vi "Initialize.vi"(8 "error in (no error)":errorcluster, 11 "GRMActor in":refnum<class "FlatFieldUI.lvclass">) -> (0 "error out":errorcluster, 3 "GRMActor out":refnum<class "FlatFieldUI.lvclass">)   [LabVIEW 2020, in "FlatField.lvlib" / "FlatFieldUI.lvlib" / "FlatFieldUI.lvclass"]
uses:
  FlatFieldUI.lvclass
  FlatField/FlatField/FlatField Status.ctl
  Displayer/Displayer/FlatField Method.ctl
  FlatFieldUI.lvclass/FlatFieldUI.ctl
  Hardware Abstraction Layer/Component/GenericActor/GenericActor/GenericController.lvclass
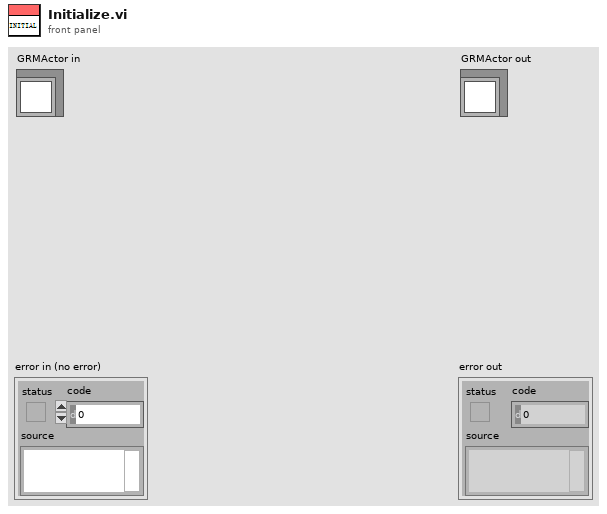
[diagram p1: front panel]
types:
  T1 = typedef "FlatField.lvlib/FlatFieldUI.lvlib/FlatFieldUI.lvclass/FlatField Method.ctl" = i32
  T2 = typedef "Image Type" = u32
  T3 = typedef "FlatField.lvlib/FlatFieldUI.lvlib/FlatFieldUI.lvclass/FlatField Status.ctl" = i32
  T4 = typedef "IMAQ Image.ctl" = refnum<image>
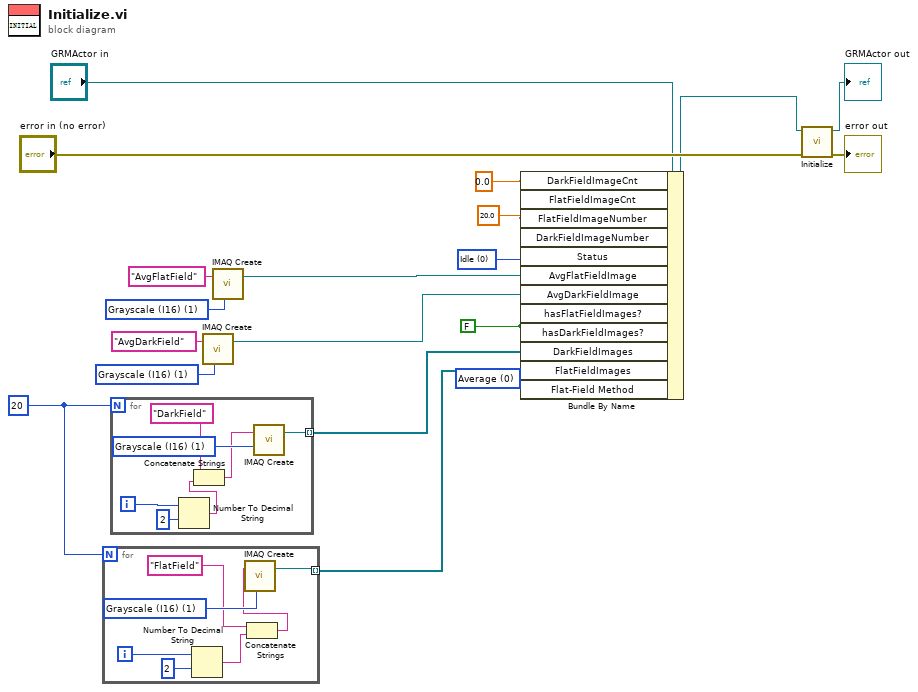
[diagram p0: block diagram]
diagram:
  w3 = T1 0 items=["Average", "Median"] ("Flat-Field Method")
  w6 = 20
  w7 = FALSE ("hasFlatFieldImages?")
  w10 = T2 1 items=["Grayscale (U8)", "Grayscale (I16)", "Grayscale (SGL)", "Complex (CSG)", "RGB (U32)", "HSL (U32)", "RGB (U64)", "Grayscale (U16)"] ("Image Type")
  w11 = T2 1 items=["Grayscale (U8)", "Grayscale (I16)", "Grayscale (SGL)", "Complex (CSG)", "RGB (U32)", "HSL (U32)", "RGB (U64)", "Grayscale (U16)"] ("Image Type")
  w14 = 0.0 ("DarkFieldImageCnt")
  w15 = 20.0 ("FieldFieldImageNumber")
  w16 = T3 0 items=["Idle", "Taking DarkField Images", "Taking FlatField Image", "Doing FlatField", ""] ("Flat-Field Status")
  n1 = for {
    N: w6 -> [_]
    tunnel: [w20] -> w4 mode=indexing
    i -> [w25]
    w26 = T2 1 items=["Grayscale (U8)", "Grayscale (I16)", "Grayscale (SGL)", "Complex (CSG)", "RGB (U32)", "HSL (U32)", "RGB (U64)", "Grayscale (U16)"] ("Image Type")
    n2 = Number To Decimal String(number=w25, width (-)=i16 2) -> (decimal integer string=w22:string)
    n3 = Concatenate Strings("FlatField" ("Image Name"), w22) -> (w21:string)
    n4 = call "IMAQ Create"("Image Name"=w21, "Image Type"=w26) -> ("New Image"=w20:T4)  [unwired: 3 in, 1 out]
  }
  n5 = for {
    N: w6 -> [_]
    tunnel: [w27] -> w5 mode=indexing
    i -> [w32]
    w33 = T2 1 items=["Grayscale (U8)", "Grayscale (I16)", "Grayscale (SGL)", "Complex (CSG)", "RGB (U32)", "HSL (U32)", "RGB (U64)", "Grayscale (U16)"] ("Image Type")
    n6 = Number To Decimal String(number=w32, width (-)=i16 2) -> (decimal integer string=w30:string)
    n7 = Concatenate Strings("DarkField" ("Image Name"), w30) -> (w28:string)
    n8 = call "IMAQ Create"("Image Name"=w28, "Image Type"=w33) -> ("New Image"=w27:T4)  [unwired: 3 in, 1 out]
  }
  n9 = call "IMAQ Create"("Image Name"="AvgDarkField", "Image Type"=w10) -> ("New Image"=w8:T4)  [unwired: 3 in, 1 out]
  n10 = call "IMAQ Create"("Image Name"="AvgFlatField", "Image Type"=w11) -> ("New Image"=w13:T4)  [unwired: 3 in, 1 out]
  n11 = Bundle By Name(cluster="GRMActor in", "DarkFieldImageCnt"=w14, "FlatFieldImageCnt"=w14, "FlatFieldImageNumber"=w15, "DarkFieldImageNumber"=w15, "Status"=w16, "AvgFlatFieldImage"=w13, "AvgDarkFieldImage"=w8, "hasFlatFieldImages?"=w7, "hasDarkFieldImages?"=w7, "DarkFieldImages"=w5, "FlatFieldImages"=w4, "Flat-Field Method"=w3) -> (w1:refnum<class "FlatFieldUI.lvclass">)
  n12 = call-parent "Initialize.vi"("error in (no error)"="error in (no error)", "GRMActor in"=w1) -> ("error out"=→"error out":errorcluster, "GRMActor out"=→"GRMActor out":refnum<class "FlatFieldUI.lvclass">)  [unwired: 8 in]
